vi "Read Excel Data.vi"(8 "error in (no error)":errorcluster, 11 "NI Generic Parser in":refnum<class "NI Generic Parser.lvclass">) -> (0 "error out":errorcluster, 2 "Excel Data":T1[](array[typedef]), 3 "NI Generic Parser out":refnum<class "NI Generic Parser.lvclass">)   [LabVIEW 2016, in "NI Generic Parser.lvlib" / "NI Generic Parser.lvclass"]
uses:
  NI Generic Parser.lvclass
  Controls/WorkSheet Data.ctl
  NI Generic Parser.lvclass/NI Generic Parser.ctl
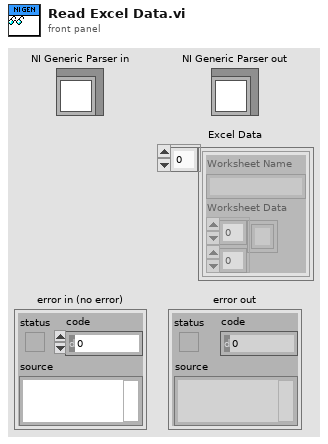
[diagram p1: front panel]
types:
  T1 = typedef "NI Generic Parser.lvlib/NI Generic Parser.lvclass/WorkSheet Data.ctl" = cluster{"Worksheet Name":string, "Worksheet Data":string[][]}
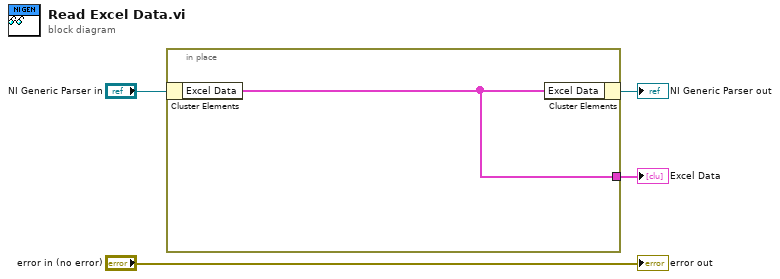
[diagram p0: block diagram]
diagram:
  n1 = in-place {
    in-place-border: [w5] -> w1
    n2 = in-place-cluster #1("NI Generic Parser in") -> ("Excel Data"=w5:T1[])
    n3 = in-place-cluster #1("Excel Data"=w5) -> (→"NI Generic Parser out":refnum<class "NI Generic Parser.lvclass">)
  }
  "Excel Data" <- w1
  "error out" <- "error in (no error)"
